vi "Confirmation Dialog.vi"(5 "Second Button Name":string="Cancel", 7 "Button Name":string="OK", 8 "error in (no error)":errorcluster, 10 "Enable":bool=TRUE) -> (0 "error out":errorcluster, 2 "Skip Prompts?":bool caption="OK", 3 "OK?":bool caption="OK", 11 "Message Display":string caption="String")   [LabVIEW 2023, in "VI Properties Editor.lvlib"]
uses:
  VI Properties Editor.lvlib
panel:
  in  "Message":string
  in  "Skip Prompts":bool caption="Don't show this message again"
  in  "Cancel":bool
  in  "OK":bool caption="OK2"
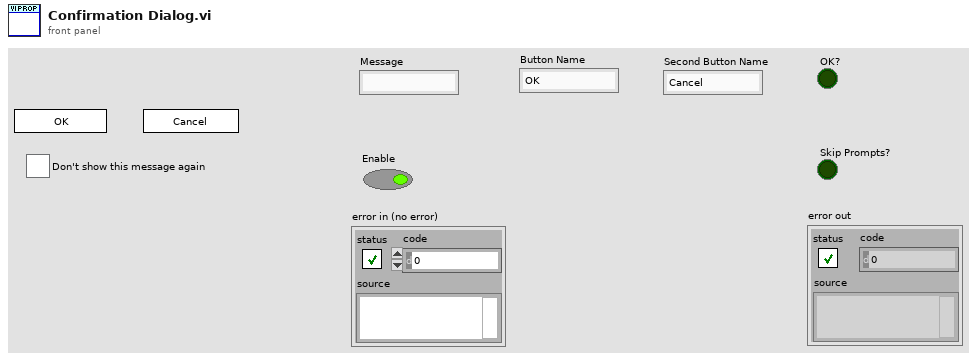
[diagram p1: front panel]
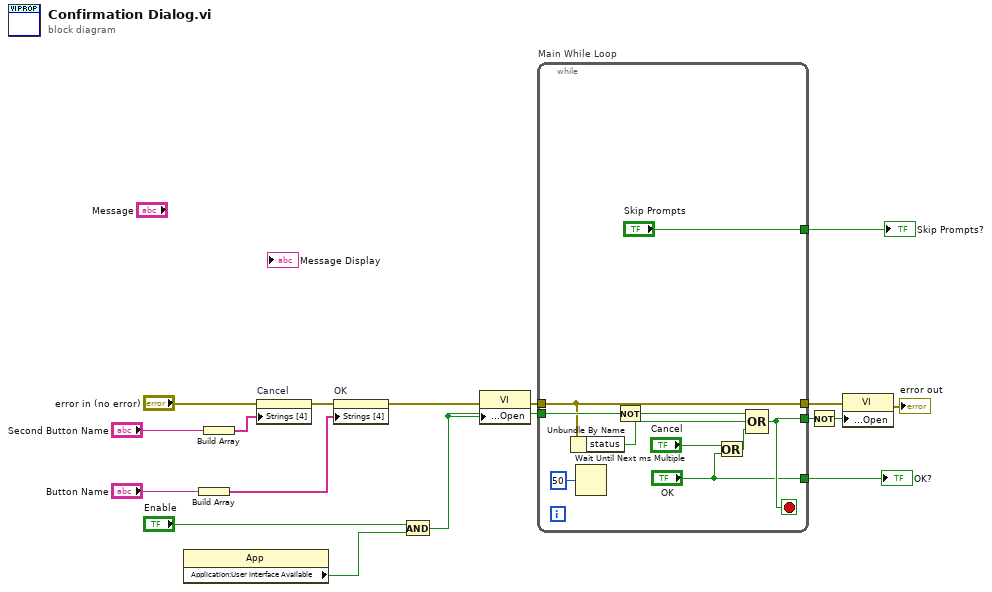
[diagram p0: block diagram]
diagram:
  n1 = property class="App"() -> ("Application:User Interface Available"=w3:bool)  [unwired: 2 in, 2 out]
  n2 = Build Array("Button Name") -> (w11:string[])
  n3 = Build Array("Second Button Name") -> (w13:string[])
  n4 = property on="Cancel" class="Bool"(error in="error in (no error)", "Strings [4]"=w13) -> (error out=w16:errorcluster)  [unwired: 1 in, 1 out]
  n5 = property on="OK" class="Bool"(error in=w16, "Strings [4]"=w11) -> (error out=w2:errorcluster)  [unwired: 1 in, 1 out]
  n6 = And(x="Enable", y=w3) -> (x .and. y?=w4:bool)
  n7 = property class="VI"(error in=w2, "Front Panel Window:Open"=w4) -> (error out=w9:errorcluster)  [unwired: 1 in, 1 out]
  n8 = while "Main While Loop" {
    tunnel: ["OK"] -> w17
    tunnel: w4 -> [w25]
    tunnel: [w23] -> w14
    tunnel: w9 -> [w22]
    tunnel: [w22] -> w7
    tunnel: ["Skip Prompts"] -> w1
    stop <- w23 stop-if-true
    n9 = Unbundle By Name(w22) -> ("status"=w20:bool)
    n10 = Wait Until Next ms Multiple(millisecond multiple=u32 50) -> ()  [unwired: 1 out]
    n11 = Not(x=w25) -> (.not. x?=w24:bool)
    n12 = Or(x="Cancel", y="OK") -> (x .or. y?=w21:bool)
    n13 = Compound Arithmetic op=OR(w24, w20, w21) -> (w23:bool)
  }
  "OK?" <- w17
  "Skip Prompts?" <- w1
  n14 = Not(x=w14) -> (.not. x?=w15:bool)
  n15 = property class="VI"(error in=w7, "Front Panel Window:Open"=w15) -> (error out=→"error out":errorcluster)  [unwired: 1 in, 1 out]
